vi "sub_daibuf_fgv.vi"(7 "cmd":enum16{"ini", "add"}(ring), 11 "data":dbl) -> (2 "mean":dbl format="%0.2f", 3 "buff":dbl[](array[numeric]))   [LabVIEW 2018]
uses:
  <vilib>/Analysis/baseanly.llb/Mean (DBL).vi
  <vilib>/Analysis/NI_AALBase.lvlib
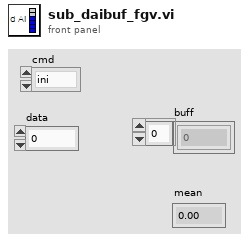
[diagram p1: front panel]
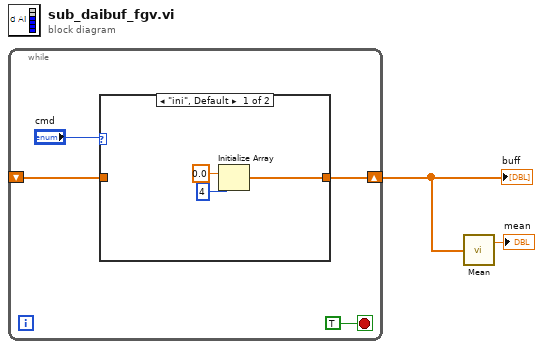
[diagram p0: block diagram]
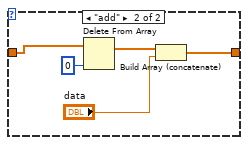
[diagram p2: hidden frame]
diagram:
  n1 = while {
    shift-right: [w4] -> w2
    shift-left: _ -> [w3]
    stop <- TRUE stop-if-true
    n2 = case shown="\"ini\", Default" "cmd" {
      tunnel: [w7 w11] -> w4
      tunnel: w3 -> [_ w12]
      frame "ini", Default {
        n3 = Initialize Array(0.0 ("element"), 4 ("dimension size")) -> (w7:dbl[])
      }
      frame "add" {
        n4 = Delete From Array(array=w12, index=0) -> (array with subset deleted=w14:dbl[])  [unwired: 1 in, 1 out]
        n5 = Build Array (concatenate)(w14, "data") -> (w11:dbl[])
      }
    }
  }
  "buff" <- w2
  n6 = call-poly <vilib>:"Mean.vi"("X"=w2) -> ("mean"=→"mean":dbl)  [unwired: 1 out]
